vi "Get Test Settings from Dictionary.vi"(8 "error in (no error)":errorcluster, 10 "name":string, 11 "TSF Parser in":refnum<class "TSF Parser.lvclass">) -> (0 "error out":errorcluster, 2 "ITestSettings Out":refnum<class "ITestSettings.lvclass">, 3 "TSF Parser out":refnum<class "TSF Parser.lvclass">)   [LabVIEW 2016, in "TSF Parser.lvlib" / "TSF Parser.lvclass"]
uses:
  TSF Parser.lvclass
  Plugins/Test Settings/ITestSettings.lvlibp/ITestSettings.lvclass
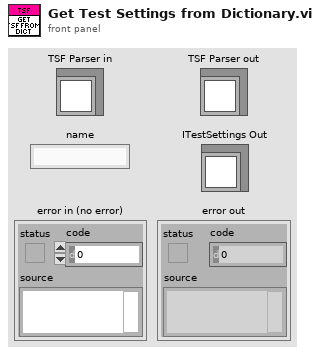
[diagram p1: front panel]
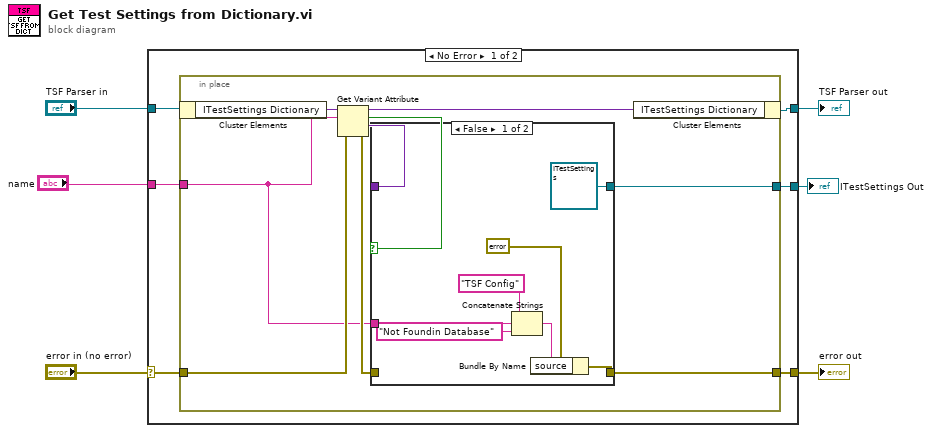
[diagram p0: block diagram]
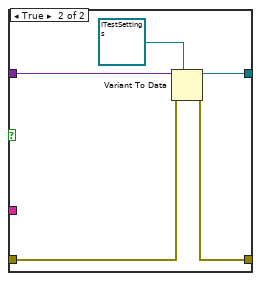
[diagram p2: hidden frame]
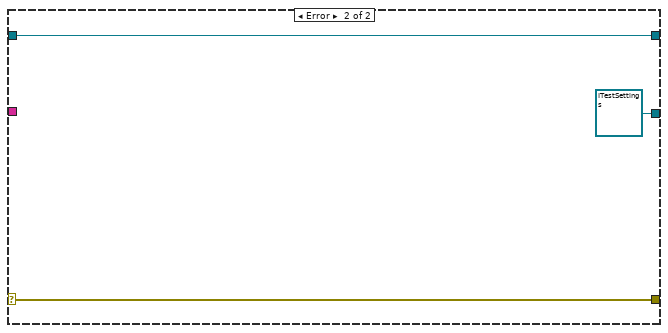
[diagram p3: hidden frame]
diagram:
  n1 = case shown="No Error" "error in (no error)" {
    selector: "error in (no error)" -> [w12 w36]
    tunnel: [w10 w36] -> w5
    tunnel: [w7 w35] -> w3
    tunnel: "TSF Parser in" -> [w11 w35]
    tunnel: "name" -> [w9 _]
    tunnel: [w8 refnum<class "ITestSettings.lvclass"> refnum ("ITestSettings.lvlibp:ITestSettings.lvclass")] -> w1
    frame No Error {
      n2 = in-place {
        in-place-border: w12 -> [w19]
        in-place-border: [w16] -> w10
        in-place-border: w9 -> [w13]
        in-place-border: [w14] -> w8
        n3 = in-place-cluster #1(w11) -> ("ITestSettings Dictionary"=w21:variant)
        n4 = Get Variant Attribute(Variant=w21, name=w13, error in=w19) -> (duplicate Variant=w20:variant, found=w15:bool, value=w18:variant, error out=w17:errorcluster)  [unwired: 1 in]
        n5 = case shown="False" w15 {
          tunnel: w18 -> [_ w33]
          tunnel: w17 -> [_ w31]
          tunnel: [w26 w30] -> w16
          tunnel: [refnum<class "ITestSettings.lvclass"> refnum ("ITestSettings.lvlibp:ITestSettings.lvclass") w29] -> w14
          tunnel: w13 -> [w24 _]
          frame False {
            n6 = Concatenate Strings("TSF Config" ("source"), w24, "Not Foundin Database" ("string")) -> (w22:string)
            n7 = Bundle By Name(cluster=errorcluster {"status"=TRUE, "code"=9904, "source"=""} ("error out"), "source"=w22) -> (w26:errorcluster)
          }
          frame True {
            n8 = Variant To Data(error in=w31, type=refnum<class "ITestSettings.lvclass"> refnum ("ITestSettings.lvlibp:ITestSettings.lvclass"), Variant=w33) -> (data=w29:refnum<class "ITestSettings.lvclass">, error out=w30:errorcluster)
          }
        }
        n9 = in-place-cluster #1("ITestSettings Dictionary"=w20) -> (w7:refnum<class "TSF Parser.lvclass">)
      }
    }
    frame Error {
    }
  }
  "error out" <- w5
  "TSF Parser out" <- w3
  "ITestSettings Out" <- w1
